vi "VITester_Provider_Interface.vi"() -> (3 "Interface Table":T1)   [LabVIEW 2013]
uses:
  <resource>/Framework/Providers/API/Provider_Interface.ctl
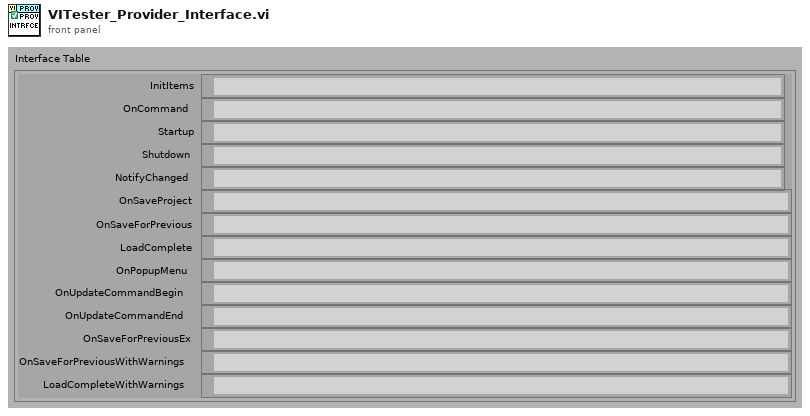
[diagram p1: front panel]
types:
  T1 = typedef "Provider_Interface.ctl" = cluster{"InitItems":path, "OnCommand":path, "Startup":path, "Shutdown":path, "NotifyChanged":path, "OnSaveProject":path, "OnSaveForPrevious":path, "LoadComplete":path, "OnPopupMenu":path, "OnUpdateCommandBegin":path, "OnUpdateCommandEnd":path, "OnSaveForPreviousEx":path, "OnSaveForPreviousWithWarnings":path, "LoadCompleteWithWarnings":path}
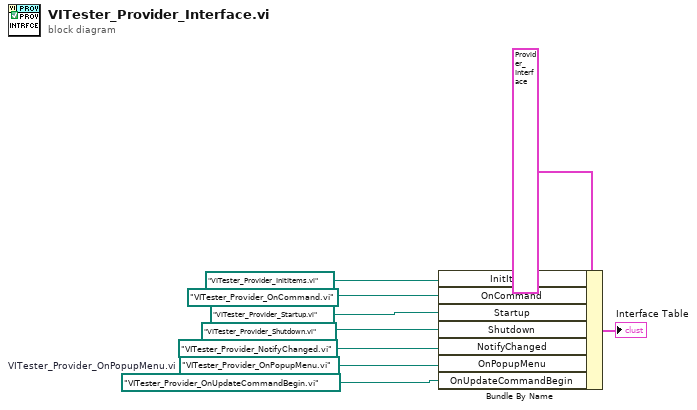
[diagram p0: block diagram]
diagram:
  w2 = path "VITester_Provider_OnPopupMenu.vi"  # VITester_Provider_OnPopupMenu.vi
  n1 = Bundle By Name(cluster=T1 {"InitItems"=path "", "OnCommand"=path "", "Startup"=path "", "Shutdown"=path "", "NotifyChanged"=path "", "OnSaveProject"=path "", "OnSaveForPrevious"=path "", "LoadComplete"=path "", "OnPopupMenu"=path "", "OnUpdateCommandBegin"=path "", "OnUpdateCommandEnd"=path "", "OnSaveForPreviousEx"=path "", "OnSaveForPreviousWithWarnings"=path "", "LoadCompleteWithWarnings"=path ""} ("InterfaceTable"), "InitItems"=path "VITester_Provider_InitItems.vi", "OnCommand"=path "VITester_Provider_OnCommand.vi", "Startup"=path "VITester_Provider_Startup.vi", "Shutdown"=path "VITester_Provider_Shutdown.vi", "NotifyChanged"=path "VITester_Provider_NotifyChanged.vi", "OnPopupMenu"=w2, "OnUpdateCommandBegin"=path "VITester_Provider_OnUpdateCommandBegin.vi") -> (→"Interface Table":T1)
